vi "Color Steps Messenger.vi"(2 "Action":T1) -> ()   [LabVIEW 2016]
uses:
  D:/Dropbox (Cambridge University)/Gurdon Lab/Edward/Microscope-Control/Microscope Modules/Color Steps/Color Steps Type Def/Color Step Actions.ctl
  D:/Dropbox (Cambridge University)/Gurdon Lab/Edward/Microscope-Control/Microscope Modules/Color Steps/Color Steps Type Def/Color Steps Notifier Type.ctl
panel:
  in  "Step":i32
  out "Current Step":i32
  out "Last Step":bool
  out "Error":errorcluster
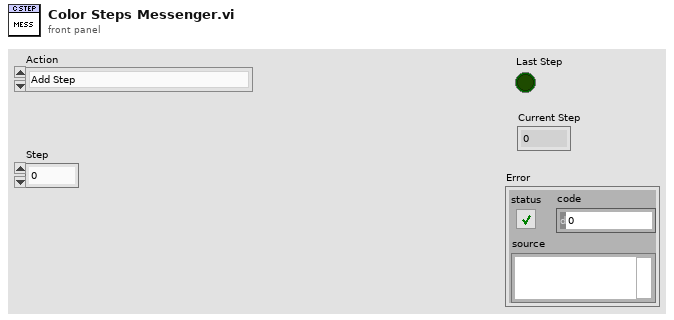
[diagram p1: front panel]
types:
  T1 = typedef "Color Step Actions.ctl" = enum16{"Add Step", "Update Step", "Remove Step", "Clear All", "Get Status", "Next Step", "Go To Step", "Save Preset", "Change Preset", "Quit"}
  T2 = typedef "Color Steps Notifier Type.ctl" = cluster{"Actions":T1, "Set Step":i32, "Current Step":i32, "Last Step?":bool, "Received?":bool, "Preset Index":i32}
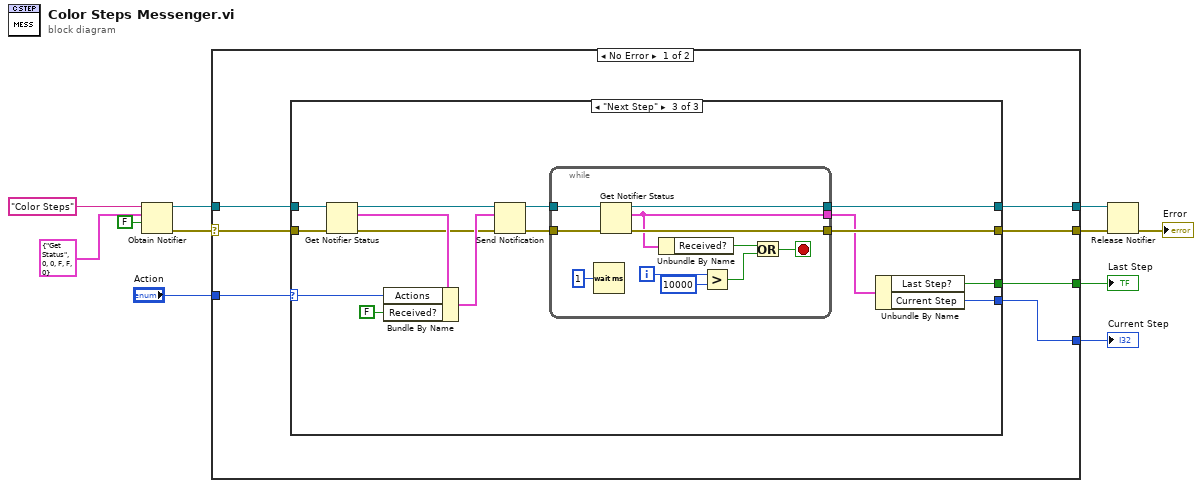
[diagram p0: block diagram]
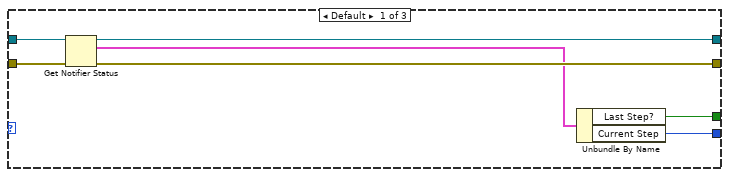
[diagram p2: hidden frame]
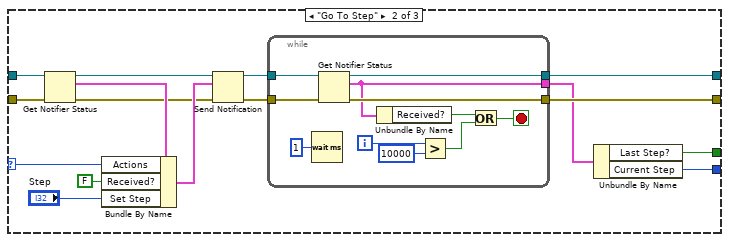
[diagram p3: hidden frame]
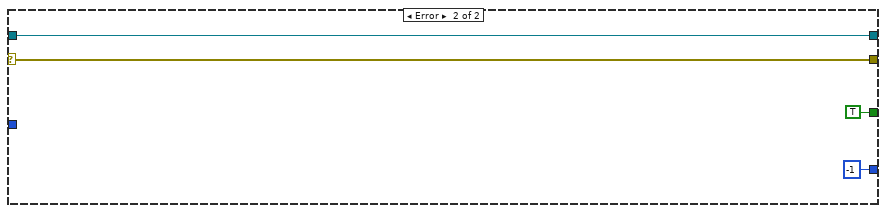
[diagram p4: hidden frame]
diagram:
  n1 = Obtain Notifier(name (unnamed)="Color Steps", notification data type=T2 {"Actions"=enum."Get Status", "Set Step"=0, "Current Step"=0, "Last Step?"=FALSE, "Received?"=FALSE, "Preset Index"=0} ("Color Steps Note Type"), create if not found? (T)=FALSE) -> (notifier out=w8:refnum<notifier>, error out=w7:errorcluster)  [unwired: 1 in, 1 out]
  n2 = case shown="No Error" w7 {
    selector: w7 -> [w15 w81]
    tunnel: w8 -> [w18 w82]
    tunnel: [w16 w82] -> w6
    tunnel: [w14 w81] -> w5
    tunnel: "Action" -> [w17 _]
    tunnel: [w13 TRUE ("Last Step?")] -> w2
    tunnel: [w12 -1 ("Current Step")] -> w1
    frame No Error {
      n3 = case shown="\"Next Step\"" w17 {
        selector: w17 -> [_ w37 w63]
        tunnel: w18 -> [w24 w41 w67]
        tunnel: [w23 w32 w59] -> w16
        tunnel: w15 -> [w25 w39 w65]
        tunnel: [w22 w30 w57] -> w14
        tunnel: [w20 w28 w55] -> w13
        tunnel: [w19 w27 w54] -> w12
        frame Default {
          n4 = Get Notifier Status(notifier=w24, error in (no error)=w25) -> (notifier out=w23:refnum<notifier>, current notification=w21:T2, error out=w22:errorcluster)  [unwired: 2 out]
          n5 = Unbundle By Name(w21) -> ("Last Step?"=w20:bool, "Current Step"=w19:i32)
        }
        frame "Go To Step" {
          n6 = Get Notifier Status(notifier=w41, error in (no error)=w39) -> (notifier out=w40:refnum<notifier>, current notification=w38:T2, error out=w26:errorcluster)  [unwired: 2 out]
          n7 = Bundle By Name(cluster=w38, "Actions"=w37, "Received?"=FALSE, "Set Step"="Step") -> (w34:T2)
          n8 = Send Notification(notification=w34, notifier=w40, error in (no error)=w26) -> (notifier out=w33:refnum<notifier>, error out=w31:errorcluster)
          n9 = while {
            tunnel: w33 -> [w52]
            tunnel: [w45] -> w32
            tunnel: w31 -> [w44]
            tunnel: [w43] -> w30
            tunnel: [w42] -> w29
            i -> [w48]
            stop <- w50 stop-if-true
            n10 = Wait (ms)(milliseconds to wait=u32 1) -> ()  [unwired: 1 out]
            n11 = Get Notifier Status(notifier=w52, error in (no error)=w44) -> (notifier out=w45:refnum<notifier>, current notification=w42:T2, error out=w43:errorcluster)  [unwired: 2 out]
            n12 = Unbundle By Name(w42) -> ("Received?"=w51:bool)
            n13 = Greater?(x=w48, y=10000) -> (0:w46:bool)
            n14 = Or(x=w51, y=w46) -> (x .or. y?=w50:bool)
          }
          n15 = Unbundle By Name(w29) -> ("Last Step?"=w28:bool, "Current Step"=w27:i32)
        }
        frame "Next Step" {
          n16 = Get Notifier Status(notifier=w67, error in (no error)=w65) -> (notifier out=w66:refnum<notifier>, current notification=w64:T2, error out=w53:errorcluster)  [unwired: 2 out]
          n17 = Bundle By Name(cluster=w64, "Actions"=w63, "Received?"=FALSE) -> (w61:T2)
          n18 = Send Notification(notification=w61, notifier=w66, error in (no error)=w53) -> (notifier out=w60:refnum<notifier>, error out=w58:errorcluster)
          n19 = while {
            tunnel: w60 -> [w78]
            tunnel: [w71] -> w59
            tunnel: w58 -> [w70]
            tunnel: [w69] -> w57
            tunnel: [w68] -> w56
            i -> [w74]
            stop <- w76 stop-if-true
            n20 = Wait (ms)(milliseconds to wait=u32 1) -> ()  [unwired: 1 out]
            n21 = Get Notifier Status(notifier=w78, error in (no error)=w70) -> (notifier out=w71:refnum<notifier>, current notification=w68:T2, error out=w69:errorcluster)  [unwired: 2 out]
            n22 = Unbundle By Name(w68) -> ("Received?"=w77:bool)
            n23 = Greater?(x=w74, y=10000) -> (0:w72:bool)
            n24 = Or(x=w77, y=w72) -> (x .or. y?=w76:bool)
          }
          n25 = Unbundle By Name(w56) -> ("Last Step?"=w55:bool, "Current Step"=w54:i32)
        }
      }
    }
    frame Error {
    }
  }
  "Last Step" <- w2
  "Current Step" <- w1
  n26 = Release Notifier(notifier=w6, error in (no error)=w5) -> (error out=→"Error":errorcluster)  [unwired: 1 in, 2 out]
